vi "WaitForMeasureComplete.vi"(8 "Error In":errorcluster, 11 "Keithley 2602 In":refnum<visa-resource-name>) -> (0 "Error Out":errorcluster, 3 "Keithley 2602 Out":refnum<visa-resource-name>)   [LabVIEW 2013]
uses:
  driver/Public/Controls/Register.ctl
  driver/Keithley-2602.lvlib
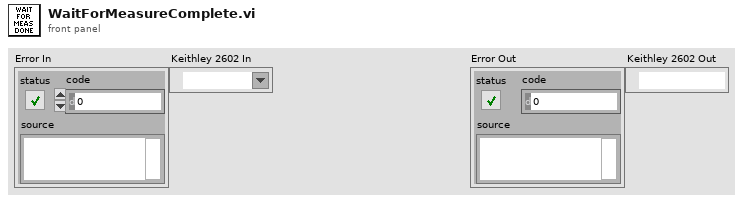
[diagram p1: front panel]
types:
  T1 = typedef "Keithley-2602.lvlib/Register.ctl" = enum16{"Condition", "Event", "Enable", "Positive Transition", "Negative Transition"}
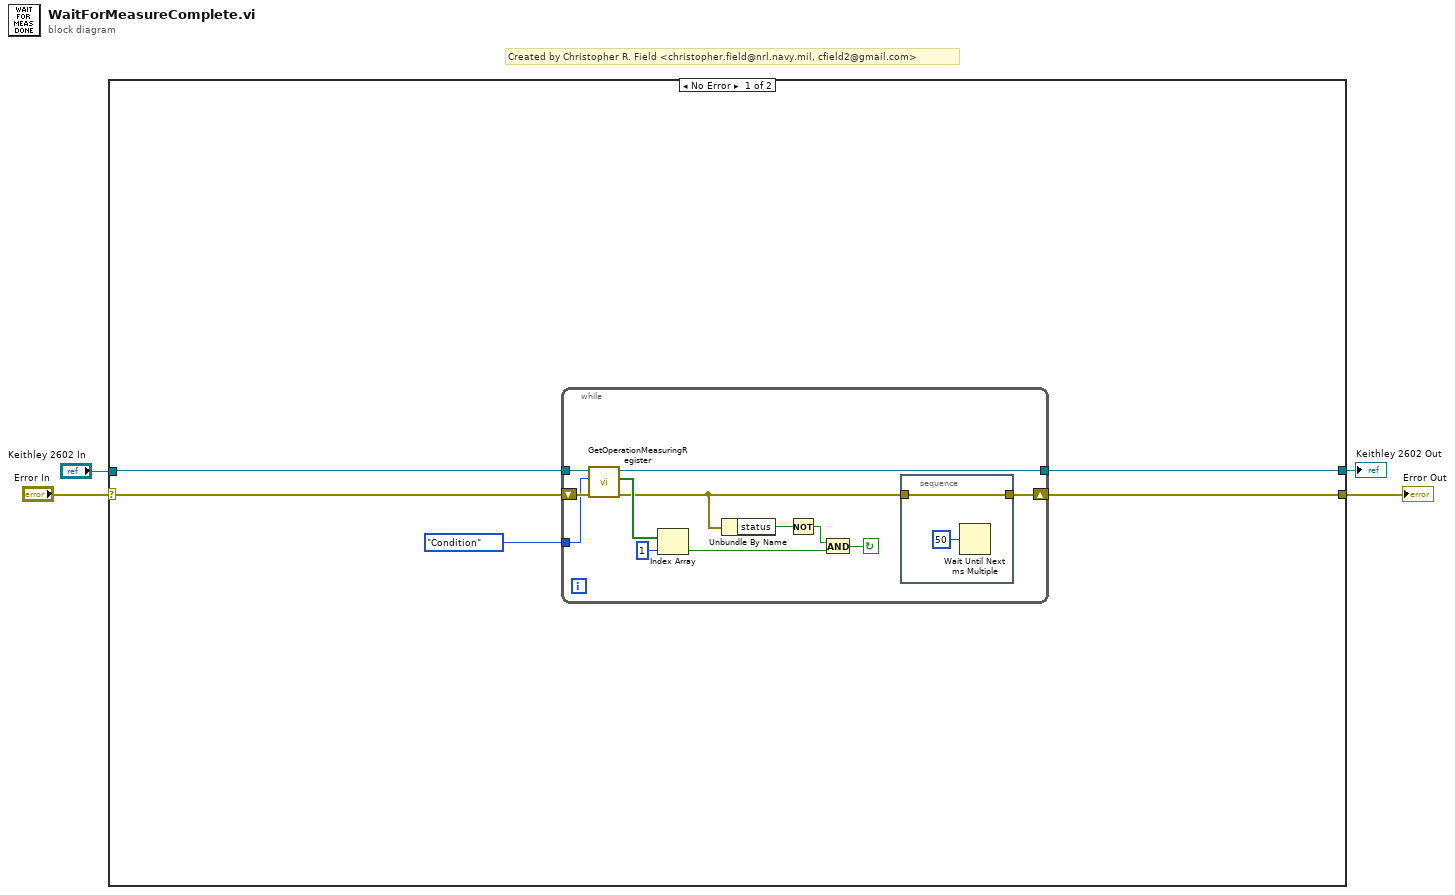
[diagram p0: block diagram]
diagram:
  # "Created by Christopher R. Field <christopher.field@nrl.navy.mil, cfield2@gmail.com>"
  n1 = case shown="No Error" "Error In" {
    selector: "Error In" -> [w8 w24]
    tunnel: "Keithley 2602 In" -> [w7 w25]
    tunnel: [w6 w25] -> w1
    tunnel: [w5 w24] -> w2
    frame No Error {
      n2 = while {
        tunnel: w7 -> [w21]
        tunnel: [w20] -> w6
        tunnel: Register."Condition" ("Register") -> [w18]
        shift-right: [w10] -> w5
        shift-left: w8 -> [w19]
        stop <- w12 continue-if-true
        n3 = call "GetOperationMeasuringRegister.vi"("Error In"=w19, "Register"=w18, "Kiethley 2602 In"=w21) -> ("Error Out"=w11:errorcluster, "Operation Measuring Register"=w17:bool[], "Keithley 2602 Out"=w20:refnum<visa-resource-name>)  [unwired: 6 in]
        n4 = Index Array(array=w17, index=1) -> (element=w15:bool)
        n5 = Unbundle By Name(w11) -> ("status"=w14:bool)
        n6 = Not(x=w14) -> (.not. x?=w13:bool)
        n7 = And(x=w13, y=w15) -> (x .and. y?=w12:bool)
        n8 = stacked-sequence {
          tunnel: w11 -> [w23]
          tunnel: [w23] -> w10
          frame #0 {
            n9 = Wait Until Next ms Multiple(millisecond multiple=u32 50) -> ()  [unwired: 1 out]
          }
        }
      }
    }
    frame Error {
    }
  }
  "Error Out" <- w2
  "Keithley 2602 Out" <- w1
